vi "Record strain.vi"() -> ()   [LabVIEW 2015]
doc: "Demonstrates the triggered peak wavelength acquisition. The peak wavelength acquisition can be untriggered, software or hardware triggered. \n\n<b>Note:</b>\nThis example is made for the instrument without channel multiplexer. Modifications will have to be made for instruments with channel multiplexer."
uses:
  Libraries/Strain/Graph.ctl
  Libraries/Strain/Micron Optics sm130/Micron Optics sm130.lvlib
panel:
  in  "Enable Unbuffered Data (Enabled)":bool=TRUE
  out "Transfer Type":u8
  out "Time delay":T1
  out "Ready":bool
  out "File":path
  out "Plots":T2
  out "Data Serial Number":u32
  out "Stored points":i32
  out "Storing data":bool
  out "Done":bool
  in  "Trigger Type (0:Untriggered)":u16(ring)=2 items=["Untriggered", "Software Triggered", "Hardware Triggered"]
  in  "Channel (1: Channel 1)":i32(ring)=1 items=["Channel 1"=1, "Channel 2"=2, "Channel 3"=3, "Channel 4"=4]
  in  "Stop":bool
  in  "Data Interleave (1)":i32=1
  in  "Number of Acquisitions (100)":i32=5000
  in  "Trigger Stop Condition (1:Edge Triggering)":u16(ring) items=["Number of Acquisitions", "Edge Triggering"]
  in  "Trigger Stop Edge (0: Rising)":u16(ring) items=["Rising", "Falling"]
  in  "Trigger Start Edge (0: Rising)":u16(ring) items=["Rising", "Falling"]
  in  "VISA resource name":refnum<visa-resource-name>="TCPIP0::192.168.1.69::1852::SOCKET"
  # "Sensor"
  # "Trigger Control"
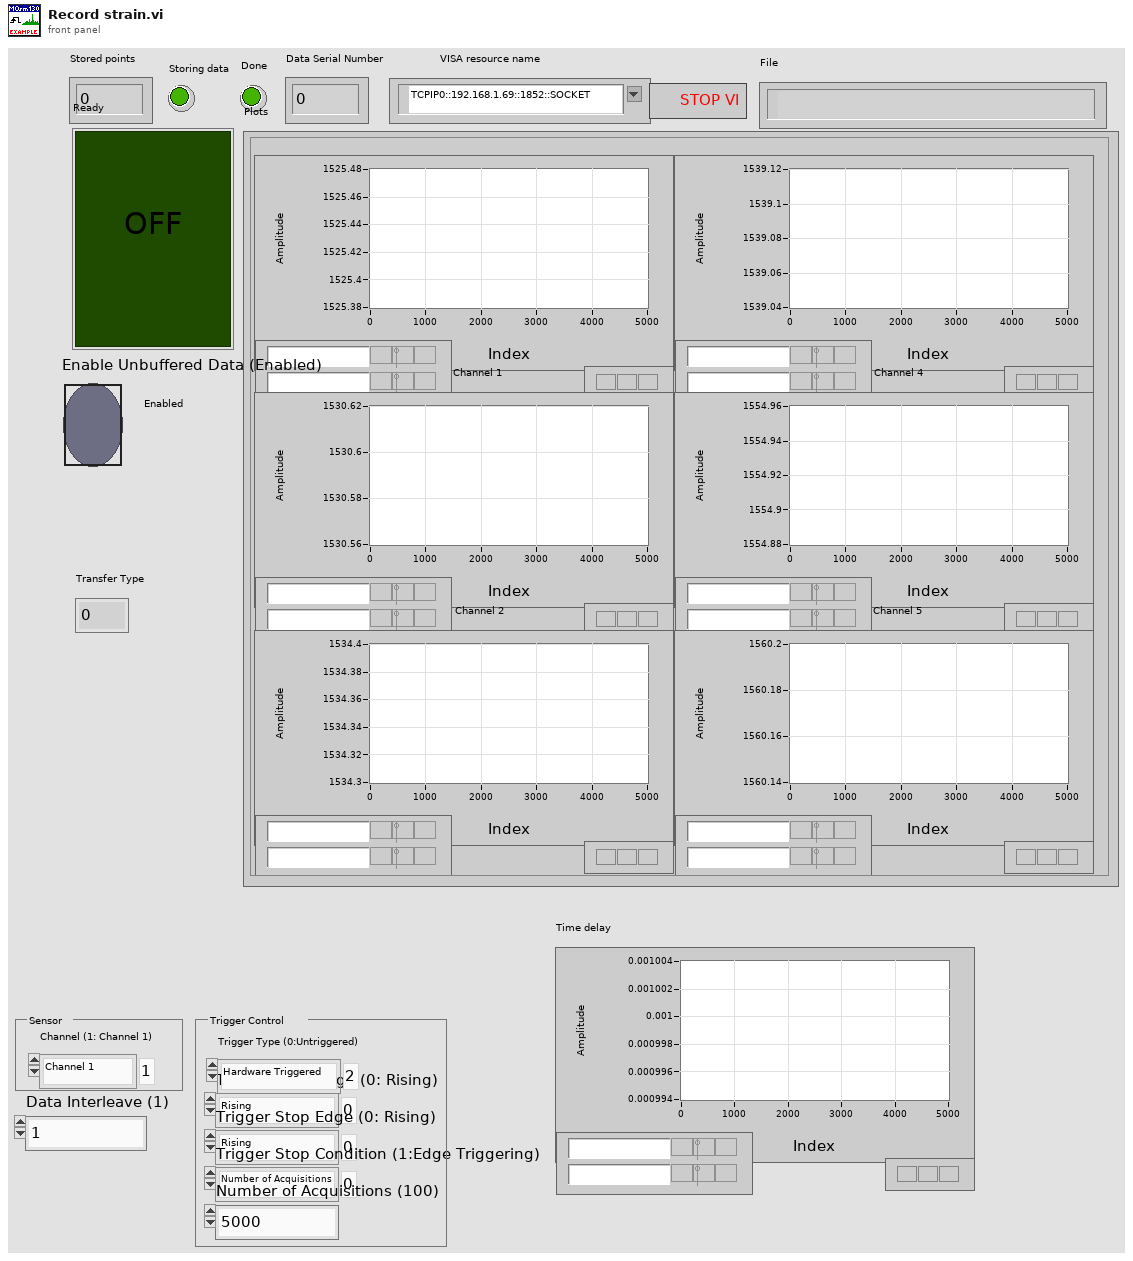
[diagram p1: front panel]
types:
  T1 = typedef "Graph.ctl" = dbl[]
  T2 = cluster{"Channel 0":T1, "Channel 1":T1, "Channel 2":T1, "Channel 3":T1, "Channel 4":T1, "Channel 5":T1}
  T3 = cluster{"Data Serial Number":u32, "Time Stamp":dbl, "Sub-Channel":u8}
  T4 = cluster{"Full Spectrum Radix":u8, "Firmware Version":u8, "Primary Fan":bool, "Secondary Fan":bool, "Switch Position":u8, "MUX":u8, "Trigger Mode":u8, "Operating Mode":u8, "Data Serial Number":u32, "Time Stamp":dbl, "Buffer (%)":u8, "MUX Level":u8}
  T5 = cluster{"Transmit Ambient Temperature":dbl, "FBG Thermistor":i16, "FFPI Peak":u16, "FBG Peak":dbl, "Kernel Src Buffer":u16, "Kernel Buffer":u16, "Kernel RT Loc0":u32, "DUT Gain":u16[], "DUT Noise Threshold":u16[], "Hardware Clock Divider":u16, "Sample Rate Divider":u16, "TEC Over Temperature":bool, "TEC Under Temperature":bool, "Transfer Type":u8}
  T6 = cluster{dbl[], dbl[], dbl[], dbl[], dbl[], dbl[]}
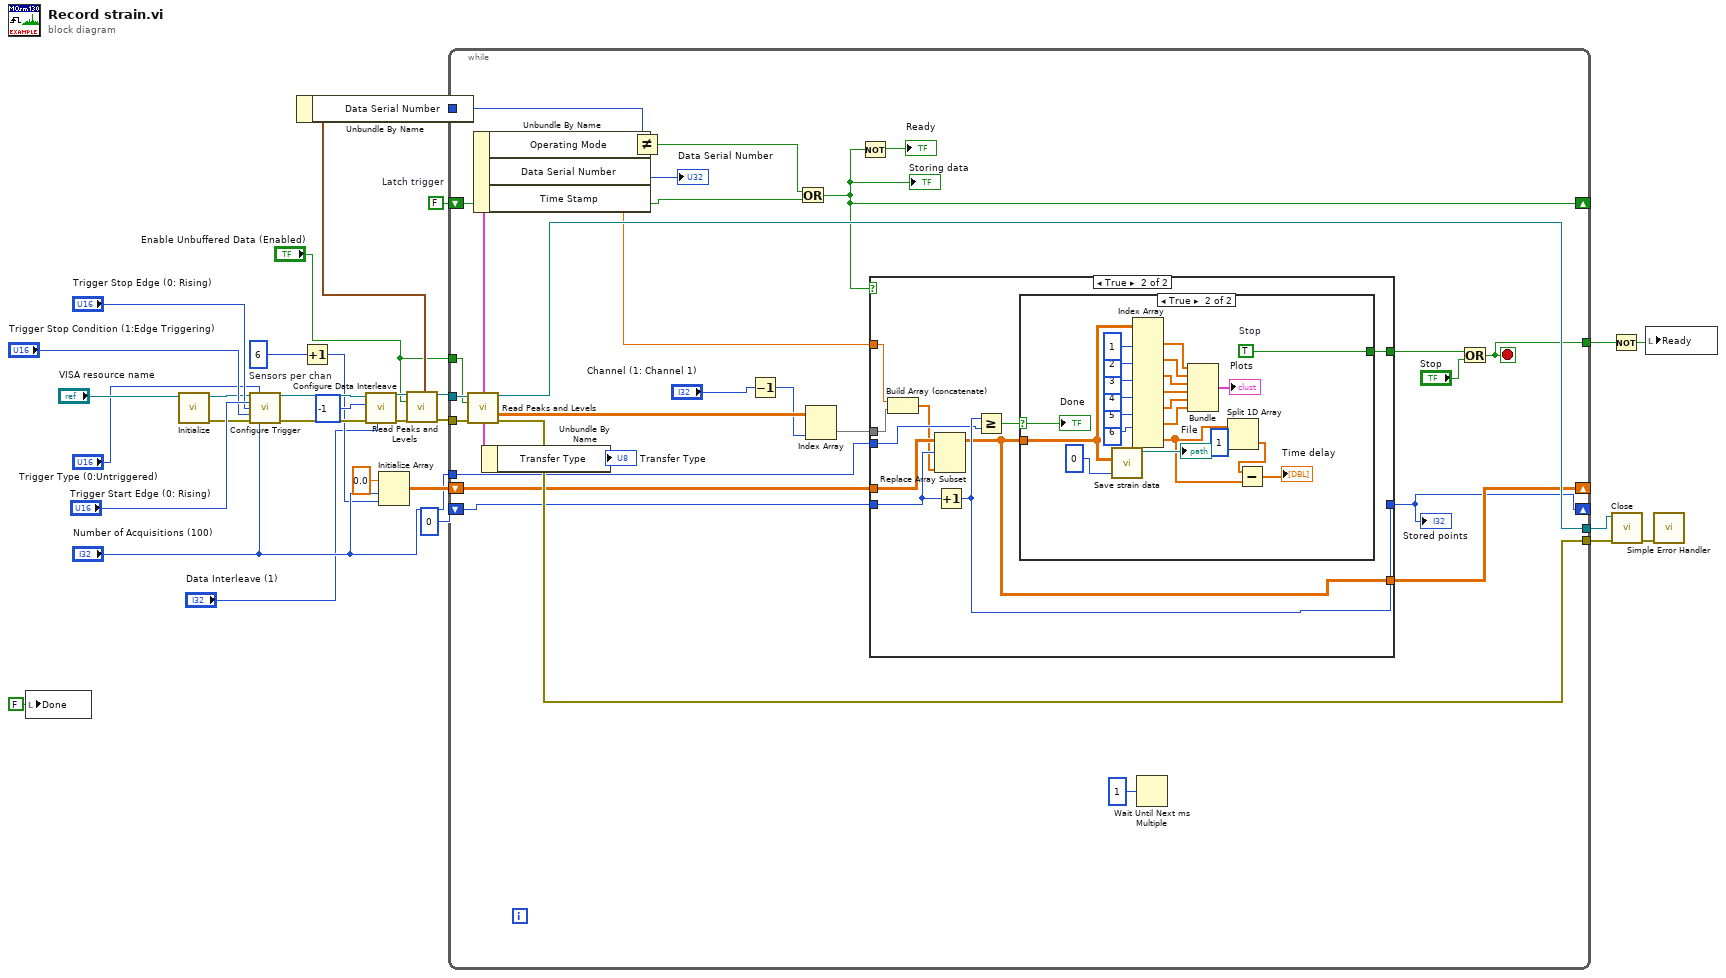
[diagram p0: block diagram]
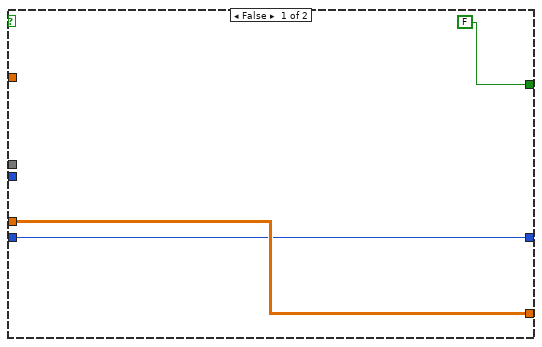
[diagram p2: hidden frame]
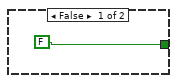
[diagram p3: hidden frame]
diagram:
  w16 = 6  # Sensors per chan
  w19 = FALSE  # Latch trigger
  n1 = local write "Done"(FALSE ("Done")) -> ()
  n2 = call "Initialize.vi"("VISA resource name"="VISA resource name") -> ("error out"=w24:errorcluster, "VISA resource name out"=w25:refnum<visa-resource-name>)  [unwired: 9 in]
  n3 = call "Configure Trigger.vi"("VISA resource name"=w25, "Trigger Type (0:Untriggered)"="Trigger Type (0:Untriggered)", "Trigger Start Edge (0: Rising)"="Trigger Start Edge (0: Rising)", "Trigger Stop Edge (0: Rising)"="Trigger Stop Edge (0: Rising)", "Trigger Stop Condition (1:Edge Triggering)"="Trigger Stop Condition (1:Edge Triggering)", "error in (no error)"=w24, "Number of Acquisitions (100)"="Number of Acquisitions (100)") -> ("VISA resource name out"=w27:refnum<visa-resource-name>, "error out"=w26:errorcluster)  [unwired: 6 in, 1 out]
  n4 = Increment(x=w16) -> (x+1=w11:i32)
  n5 = call "Configure Data Interleave.vi"("Data Interleave (1)"="Data Interleave (1)", "error in (no error)"=w26, "Sensor Number (1)"=-1, "VISA resource name"=w27) -> ("error out"=w8:errorcluster, "VISA resource name out"=w5:refnum<visa-resource-name>)  [unwired: 6 in]
  n6 = Initialize Array(0.0 ("element"), "Number of Acquisitions (100)", w11) -> (w17:dbl[][])
  n7 = call "Read Peaks and Levels.vi"("VISA resource name"=w5, "Enable Unbuffered Data (Enabled)"="Enable Unbuffered Data (Enabled)", "error in (no error)"=w8) -> ("Data Status"=w4:T3, "VISA resource name out"=w6:refnum<visa-resource-name>, "error out"=w7:errorcluster)  [unwired: 4 in, 6 out]
  n8 = Unbundle By Name(w4) -> ("Data Serial Number"=w3:u32)
  n9 = while {
    tunnel: w6 -> [w48]
    tunnel: w7 -> [w49]
    tunnel: [w57] -> w22
    tunnel: [w56] -> w21
    shift-right: [w40] -> _
    shift-left: w19 -> [w41]
    shift-right: [w53] -> _
    shift-left: w17 -> [w55]
    shift-right: [w47] -> _
    shift-left: 0 -> [w54]
    tunnel: "Number of Acquisitions (100)" -> [w52]
    tunnel: [w39] -> w9
    tunnel: w3 -> [w38]
    tunnel: "Enable Unbuffered Data (Enabled)" -> [w32]
    stop <- w39 stop-if-true
    n10 = call "Read Peaks and Levels.vi"("VISA resource name"=w48, "Enable Unbuffered Data (Enabled)"=w32, "error in (no error)"=w49) -> ("Status"=w35:T4, "VISA resource name out"=w57:refnum<visa-resource-name>, "Peak Wavelengths (nm)"=w46:dbl[][], "Reserved"=w34:T5, "error out"=w56:errorcluster)  [unwired: 4 in, 4 out]
    n11 = Unbundle By Name(w35) -> ("Data Serial Number"=w36:u32, "Time Stamp"=w42:dbl)  [unwired: 1 out]
    "Data Serial Number" <- w36
    n12 = Unbundle By Name(w34) -> ("Transfer Type"=→"Transfer Type":u8)
    n13 = Not Equal?(x=w38, y=w36) -> (x != y?=w37:bool)
    n14 = Decrement(x="Channel (1: Channel 1)") -> (x-1=w44:i32)
    n15 = Or(x=w37, y=w41) -> (x .or. y?=w40:bool)
    "Storing data" <- w40
    n16 = Index Array(array=w46, index (col)=w44) -> (element=w45:dbl[])  [unwired: 1 in]
    n17 = Not(x=w40) -> (.not. x?=→"Ready":bool)
    n18 = case shown="True" w40 {
      tunnel: w55 -> [w62 w72]
      tunnel: w45 -> [_ w71]
      tunnel: [w61 w70] -> w47
      tunnel: w54 -> [w61 w65]
      tunnel: [w62 w67] -> w53
      tunnel: w52 -> [_ w69]
      tunnel: [FALSE w66] -> w50
      tunnel: w42 -> [_ w63]
      frame False {
      }
      frame True {
        n19 = Build Array (concatenate)(w63, w71) -> (w64:dbl[])
        n20 = Replace Array Subset(array=w72, new element=w64, index (row)=w65) -> (w67:dbl[][])  [unwired: 1 in]
        n21 = Increment(x=w65) -> (x+1=w70:i32)
        n22 = Greater Or Equal?(x=w70, y=w69) -> (x >= y?=w68:bool)
        n23 = case shown="True" w68 {
          selector: w68 -> [_ w95]
          tunnel: w67 -> [_ w93]
          tunnel: [FALSE w94] -> w66
          frame False {
          }
          frame True {
            w94 = TRUE  # Stop
            n24 = call "Save strain data.vi"("Data"=w93) -> ("File name"=→"File":path)  [unwired: 9 in, 1 out]
            n25 = Index Array(array=w93, index (col) #1=1 ("index (row)"), index (col) #2=2 ("index (row)"), index (col) #3=3 ("index (row)"), index (col) #4=4 ("index (row)"), index (col) #5=5 ("index (row)"), index (col) #6=6 ("index (row)"), index (col) #7=0 ("index (row)")) -> (element #1=w92:dbl[], element #2=w91:dbl[], element #3=w90:dbl[], element #4=w89:dbl[], element #5=w88:dbl[], element #6=w87:dbl[], element #7=w75:dbl[])  [unwired: 7 in]
            n26 = Bundle(w92, w91, w90, w89, w88, w87) -> (→"Plots":T6)  [unwired: 1 in]
            n27 = Split 1D Array(array=w75, index=1) -> (second subarray=w76:dbl[])  [unwired: 1 out]
            n28 = Subtract(x=w76, y=w75) -> (x-y=→"Time delay":dbl[])
            "Done" <- w95
          }
        }
      }
    }
    "Stored points" <- w47
    n29 = Wait Until Next ms Multiple(millisecond multiple=u32 1) -> ()  [unwired: 1 out]
    n30 = Or(x=w50, y="Stop") -> (x .or. y?=w39:bool)
  }
  n31 = Not(x=w9) -> (.not. x?=w10:bool)
  n32 = call "Close.vi"("error in (no error)"=w21, "VISA resource name"=w22) -> ("error out"=w20:errorcluster)  [unwired: 9 in]
  n33 = local write "Ready"(w10) -> ()
  n34 = call <vilib>:"Simple Error Handler.vi"("error in (no error)"=w20) -> ()  [unwired: 4 in, 5 out]
